vi "subscribe.vi"(7 "QoS":T1, 8 "error in":errorcluster, 10 "topic":string, 11 "MQTT client in":refnum<class "MQTT client.lvclass">) -> (0 "error out":errorcluster, 2 "request ID":i32, 3 "MQTT client out":refnum<class "MQTT client.lvclass">)   [LabVIEW 2014, in "MQTT client.lvclass"]
uses:
  MQTT client.lvclass
  QoS levels.ctl
  MQTT client.lvclass/MQTT client.ctl
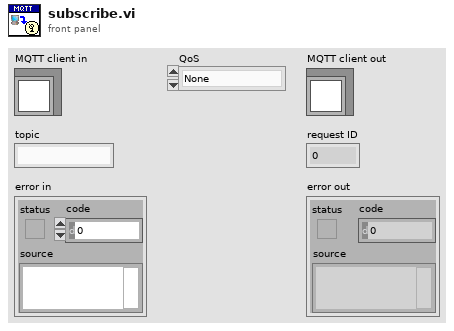
[diagram p1: front panel]
types:
  T1 = typedef "MQTT client.lvclass/QoS levels.ctl" = enum8{"None", "At least once", "Exactly once"}
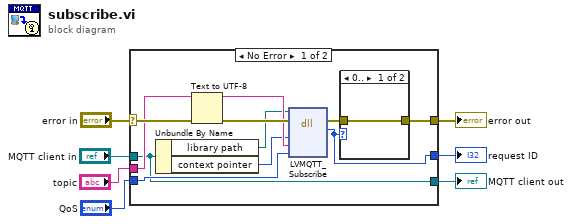
[diagram p0: block diagram]
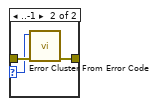
[diagram p2: hidden frame]
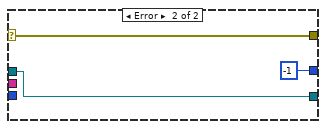
[diagram p3: hidden frame]
diagram:
  n1 = case shown="No Error" "error in" {
    selector: "error in" -> [w13 w25]
    tunnel: [w15 w25] -> w6
    tunnel: [w10 w24] -> w4
    tunnel: "MQTT client in" -> [w10 w24]
    tunnel: [w14 -1 ("return type")] -> w3
    tunnel: "QoS" -> [w12 _]
    tunnel: "topic" -> [w11 _]
    frame No Error {
      n2 = Unbundle By Name(w10) -> ("library path"=w8:path, "context pointer"=w9:u64)
      n3 = Text to UTF-8(8:w13, 11:w11) -> (0:w18:errorcluster, 3:w17:string)  [unwired: 1 in]
      n4 = dll-call lib="paho-mqtt3a.dll" fn="LVMQTT_Subscribe"(path in=w8, error in=w18, "lvctx"=w9, "topic"=w17, "qos"=w12) -> (error out=w16:errorcluster, "return type"=w14:i32)  [unwired: 4 in, 1 out]
      n5 = case shown="0.." w14 {
        selector: w14 -> [_ w20]
        tunnel: w16 -> [w19 w22]
        tunnel: [w19 w21] -> w15
        frame 0.. {
        }
        frame ..-1 {
          n6 = call <vilib>:"Error Cluster From Error Code.vi"("error in (no error)"=w22, "error code (0)"=w20) -> ("error out"=w21:errorcluster)  [unwired: 7 in]
        }
      }
    }
    frame Error {
    }
  }
  "error out" <- w6
  "MQTT client out" <- w4
  "request ID" <- w3
